vi "test.Launcher(singleEvent).vi"() -> ()   [LabVIEW 2017, in "TimerEngine.lvlib"]
uses:
  TimerEngine.lvlib
  TimerEngine.lvclass
panel:
  out "Timer":string
  out "Status.Start?":bool
  out "Status.TimePeroid(ms)":i64
  out "Status.EclipsedTime(ms)":i64
  out "diff 2(ms)":dbl(graph)
  out "diff 1(ms) history":dbl(graph)
  in  "rename timer1":bool
  out "ready?":bool
  in  "enable 2":bool=TRUE
  in  "enable 1":bool=TRUE
  out "diff 1(ms)":dbl
  out "diff 2(ms)":dbl
  in  "TimePeroid(ms)":i32=1000
  out "Timer Descriptions":string[](array[string])
  in  "unregister timer1":bool
  in  "unregister timer2":bool
  out "[current time]":timestamp
  out "current time 2":timestamp
  out "Event Time Stamp 2":timestamp
  out "Event Time Stamp":timestamp
  out "current time":timestamp
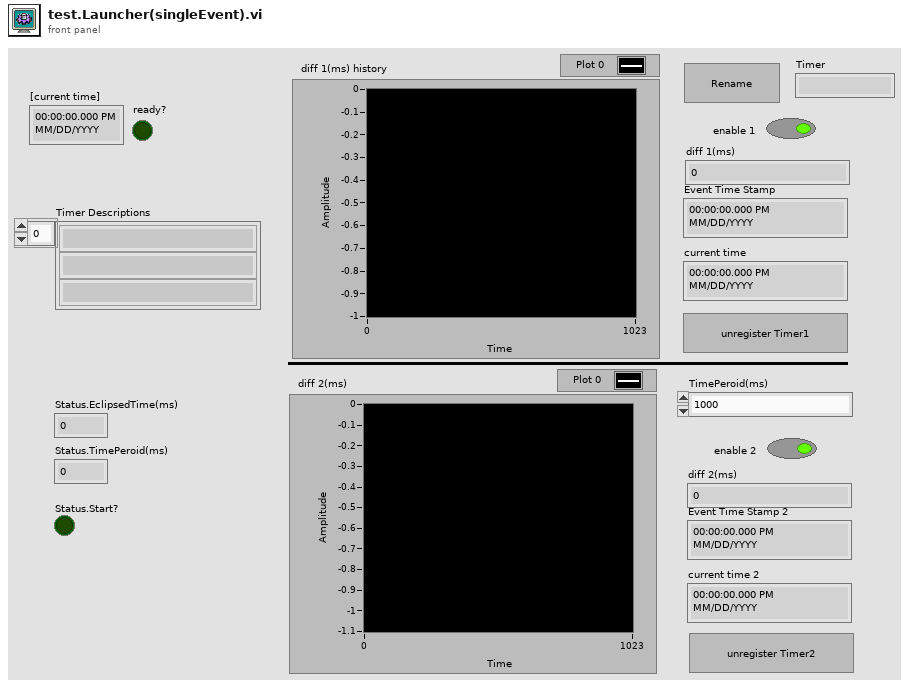
[diagram p1: front panel]
types:
  T1 = typedef "TimerEngine.lvlib/TimerEngine.lvclass/Timer-UserEvent.ctl" = refnum<user-event>
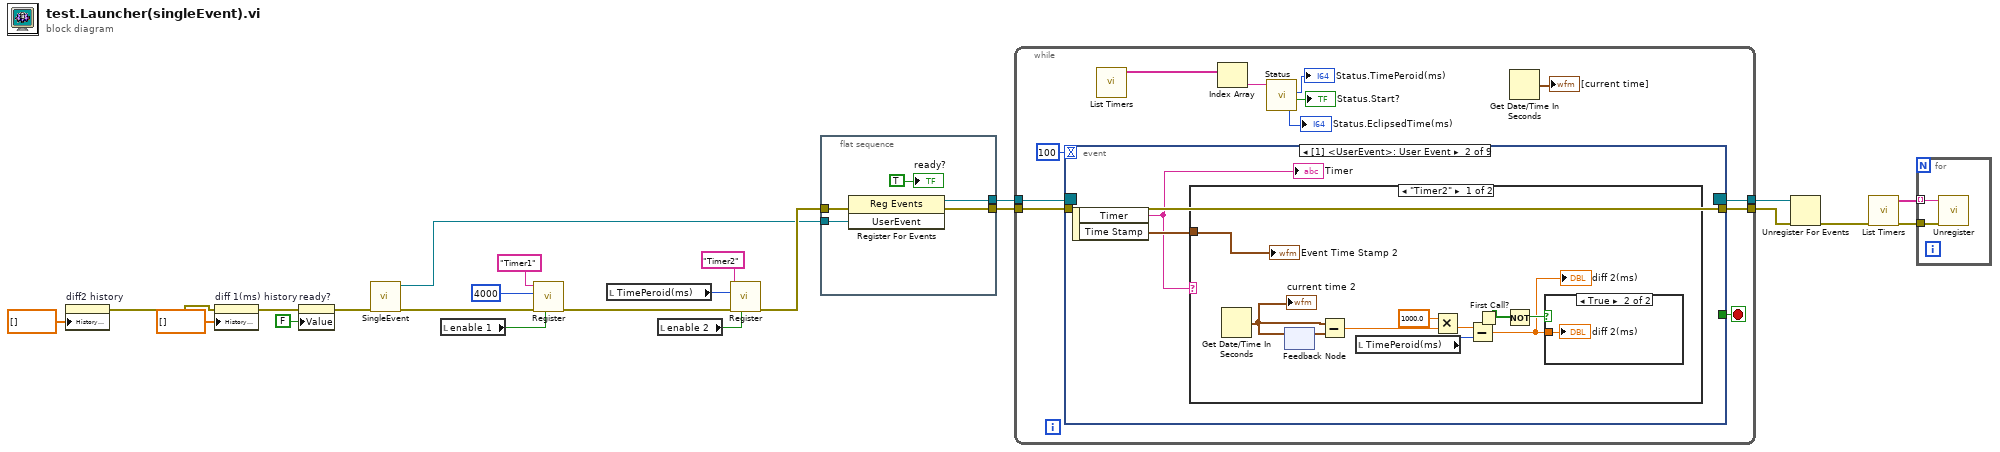
[diagram p0: block diagram]
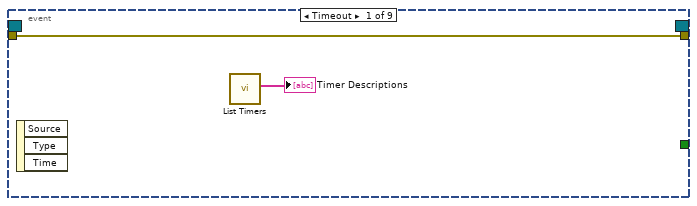
[diagram p2: hidden frame]
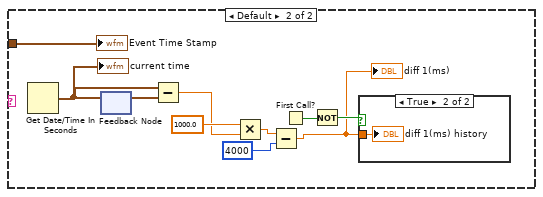
[diagram p4: hidden frame]
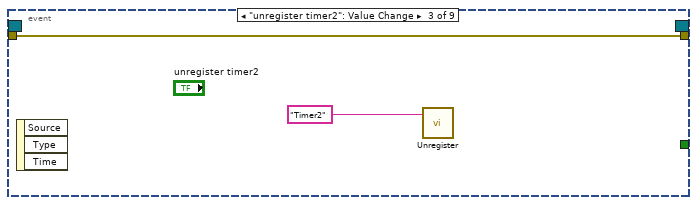
[diagram p6: hidden frame]
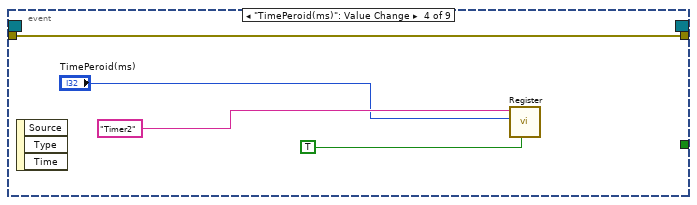
[diagram p7: hidden frame]
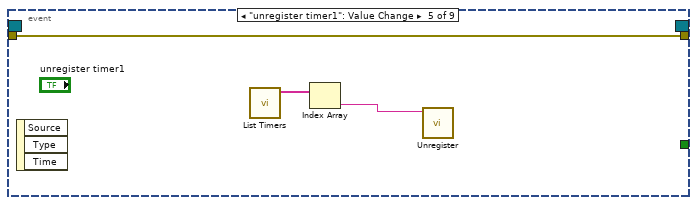
[diagram p8: hidden frame]
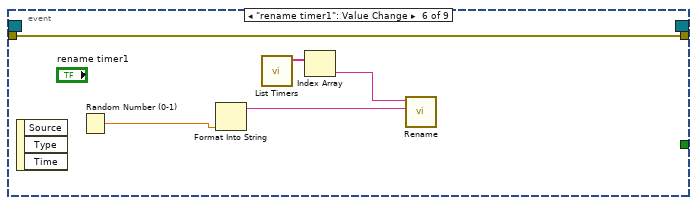
[diagram p9: hidden frame]
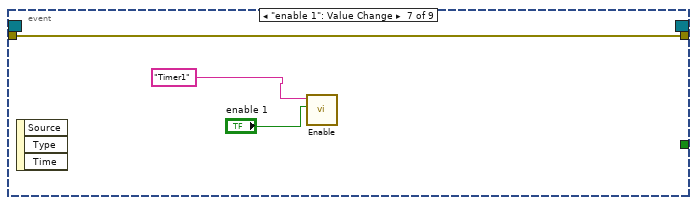
[diagram p10: hidden frame]
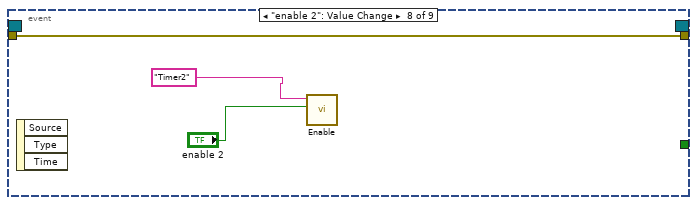
[diagram p11: hidden frame]
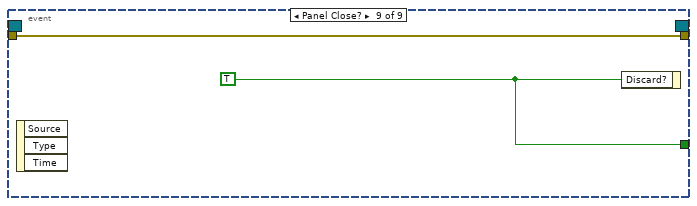
[diagram p12: hidden frame]
diagram:
  n1 = property on="diff2 history" class="WFChart (strict)"("History Data"=dbl[] []) -> (error out=w3:errorcluster)  [unwired: 2 in, 1 out]
  n2 = property on="diff 1(ms) history" class="WFChart (strict)"(error in=w3, "History Data"=dbl[] []) -> (error out=w5:errorcluster)  [unwired: 1 in, 1 out]
  n3 = property on="ready?" class="Bool (strict)"(error in=w5, "Value"=FALSE ("ready?")) -> (error out=w10:errorcluster)  [unwired: 1 in, 1 out]
  n4 = call "SingleEvent.vi"("error in (no error)"=w10) -> ("error out"=w2:errorcluster, "UserEvent"=w1:T1)  [unwired: 9 in]
  n5 = local read "enable 1"() -> (w13:bool)
  n6 = call "Register.vi"("Start Imidiatlely?(T)"=w13, "error in (no error)"=w2, "TimePeroid(ms)"=4000, "Name"="Timer1") -> ("error out"=w17:errorcluster)  [unwired: 6 in, 1 out]
  n7 = local read "TimePeroid(ms)"() -> (w14:i32)
  n8 = local read "enable 2"() -> (w12:bool)
  n9 = call "Register.vi"("Start Imidiatlely?(T)"=w12, "error in (no error)"=w17, "TimePeroid(ms)"=w14, "Name"="Timer2") -> ("error out"=w15:errorcluster)  [unwired: 6 in, 1 out]
  n10 = flat-sequence {
    tunnel: [w28] -> w22
    tunnel: [w27] -> w20
    tunnel: w15 -> [w26]
    tunnel: w1 -> [w24]
    frame #0 {
      n11 = register-events(error in=w26, w24) -> (reference out=w28:refnum<event-registration>, error out=w27:errorcluster)  [unwired: 1 in]
      "ready?" <- TRUE ("ready?")
    }
  }
  n12 = while {
    tunnel: w22 -> [w40]
    tunnel: [w38] -> w21
    tunnel: w20 -> [w37]
    tunnel: [w36] -> w19
    stop <- w39 stop-if-true
    n13 = event shown="[1] <UserEvent>: User Event" {
      selector: w40 -> [_ _ _ _ _ _ _ _ _]
      dyn-events: [_ _ _ _ _ _ _ _ _] -> w38
      timeout: 100 -> [_ _ _ _ _ _ _ _ _]
      tunnel: [_ _ _ _ _ _ _ _ w89] -> w39
      tunnel: w37 -> [w42 w45 w69 w73 w76 w81 w84 w87 w88]
      tunnel: [w42 w45 w69 w73 w76 w81 w84 w87 w88] -> w36
      event Timeout {
        n14 = event-data() -> ()  [unwired: 1 in, 3 out]
        n15 = call "List Timers.vi"() -> ("Timer Descriptions"=→"Timer Descriptions":string[])  [unwired: 9 in, 2 out]
      }
      event User Event {
        n16 = event-data() -> ("Timer"=w43:string, "Time Stamp"=w44:timestamp)  [unwired: 1 in]
        "Timer" <- w43
        n17 = case shown="\"Timer2\"" w43 {
          tunnel: w44 -> [w46 w66]
          frame "Timer2" {
            n18 = Get Date/Time In Seconds() -> (seconds since 1Jan1904=w55:timestamp)
            "current time 2" <- w55
            n19 = feedback #1() -> (w54:timestamp)  [unwired: 1 in]
            n20 = feedback-in #1(w55) -> ()
            n21 = Subtract(x=w55, y=w54) -> (x-y=w51:dbl)
            n22 = local read "TimePeroid(ms)"() -> (w50:i32)
            n23 = Multiply(x=1000.0, y=w51) -> (x*y=w49:dbl)
            n24 = Subtract(x=w49, y=w50) -> (x-y=w48:dbl)
            "diff 2(ms)" <- w48
            n25 = First Call?() -> (First Call?: T/F=w52:bool)
            n26 = Not(x=w52) -> (.not. x?=w53:bool)
            n27 = case shown="True" w53 {
              tunnel: w48 -> [_ w56]
              frame False {
              }
              frame True {
                "diff 2(ms)" <- w56
              }
            }
            "Event Time Stamp 2" <- w46
          }
          frame Default {
            n28 = Get Date/Time In Seconds() -> (seconds since 1Jan1904=w64:timestamp)
            "current time" <- w64
            n29 = feedback #2() -> (w65:timestamp)  [unwired: 1 in]
            n30 = feedback-in #2(w64) -> ()
            n31 = Subtract(x=w64, y=w65) -> (x-y=w60:dbl)
            n32 = Multiply(x=1000.0, y=w60) -> (x*y=w59:dbl)
            n33 = Subtract(x=w59, y=4000 ("TimePeroid(ms)")) -> (x-y=w57:dbl)
            "diff 1(ms)" <- w57
            n34 = First Call?() -> (First Call?: T/F=w63:bool)
            n35 = Not(x=w63) -> (.not. x?=w62:bool)
            n36 = case shown="True" w62 {
              tunnel: w57 -> [_ w67]
              frame False {
              }
              frame True {
                "diff 1(ms) history" <- w67
              }
            }
            "Event Time Stamp" <- w66
          }
        }
      }
      event "unregister timer2": Value Change {
        n37 = event-data() -> ()  [unwired: 1 in, 3 out]
        n38 = call "Unregister.vi"("Name"="Timer2") -> ()  [unwired: 10 in, 1 out]
      }
      event "TimePeroid(ms)": Value Change {
        n39 = event-data() -> ()  [unwired: 1 in, 3 out]
        n40 = call "Register.vi"("Start Imidiatlely?(T)"=TRUE ("Start Imidiatlely?(F)"), "TimePeroid(ms)"="TimePeroid(ms)", "Name"="Timer2") -> ()  [unwired: 7 in, 2 out]
      }
      event "unregister timer1": Value Change {
        n41 = event-data() -> ()  [unwired: 1 in, 3 out]
        n42 = call "List Timers.vi"() -> ("Timers"=w75:string[])  [unwired: 9 in, 2 out]
        n43 = Index Array(array=w75) -> (element=w74:string)  [unwired: 1 in]
        n44 = call "Unregister.vi"("Name"=w74) -> ()  [unwired: 10 in, 1 out]
      }
      event "rename timer1": Value Change {
        n45 = event-data() -> ()  [unwired: 1 in, 3 out]
        n46 = Random Number (0-1)() -> (number: 0 to 1=w80:dbl)
        n47 = Format Into String(w80) -> (resulting string=w79:string)  [unwired: 3 in, 1 out]
        n48 = call "List Timers.vi"() -> ("Timers"=w78:string[])  [unwired: 9 in, 2 out]
        n49 = Index Array(array=w78) -> (element=w77:string)  [unwired: 1 in]
        n50 = call "Rename.vi"("New Name"=w79, "Name"=w77) -> ()  [unwired: 9 in, 1 out]
      }
      event "enable 1": Value Change {
        n51 = event-data() -> ()  [unwired: 1 in, 3 out]
        n52 = call "Enable.vi"("Enable?"="enable 1", "Name"="Timer1") -> ()  [unwired: 9 in, 1 out]
      }
      event "enable 2": Value Change {
        n53 = event-data() -> ()  [unwired: 1 in, 3 out]
        n54 = call "Enable.vi"("Enable?"="enable 2", "Name"="Timer2") -> ()  [unwired: 9 in, 1 out]
      }
      event Panel Close? {
        w89 = TRUE ("Discard?")
        n55 = event-data() -> ()  [unwired: 1 in, 3 out]
        n56 = event-data("Discard?"=w89) -> ()  [unwired: 1 in, 1 out]
      }
    }
    n57 = call "List Timers.vi"() -> ("Timers"=w33:string[])  [unwired: 9 in, 2 out]
    n58 = Index Array(array=w33) -> (element=w32:string)  [unwired: 1 in]
    n59 = call "Status.vi"("Name"=w32) -> ("Start?"=→"Status.Start?":bool, "TimePeroid(ms)"=→"Status.TimePeroid(ms)":i64, "EclipsedTime(ms)"=→"Status.EclipsedTime(ms)":i64)  [unwired: 6 in, 2 out]
    n60 = Get Date/Time In Seconds() -> (seconds since 1Jan1904=→"[current time]":timestamp)
  }
  n61 = Unregister For Events(event registration refnum=w21, error in=w19) -> (error out=w18:errorcluster)
  n62 = call "List Timers.vi"("error in (no error)"=w18) -> ("error out"=w8:errorcluster, "Timers"=w7:string[])  [unwired: 8 in, 1 out]
  n63 = for {
    tunnel: w8 -> [w91]
    tunnel: w7 -> [w90] mode=indexing
    n64 = call "Unregister.vi"("error in (no error)"=w91, "Name"=w90) -> ()  [unwired: 9 in, 1 out]
  }
